vi "Detect Phase.vi"(11 "Input Wavceform":waveform(i16)) -> (1 "Phase in Degress":dbl, 2 "Phase in Samples":dbl, 3 "Detected Sine Frequency":dbl format="%.2p")   [LabVIEW 2011]
uses:
  <vilib>/measure/matone.llb/Extract Single Tone Information 1 Chan.vi
  <vilib>/measure/NI_MAPro.lvlib
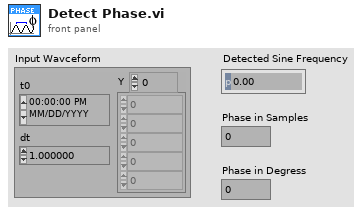
[diagram p1: front panel]
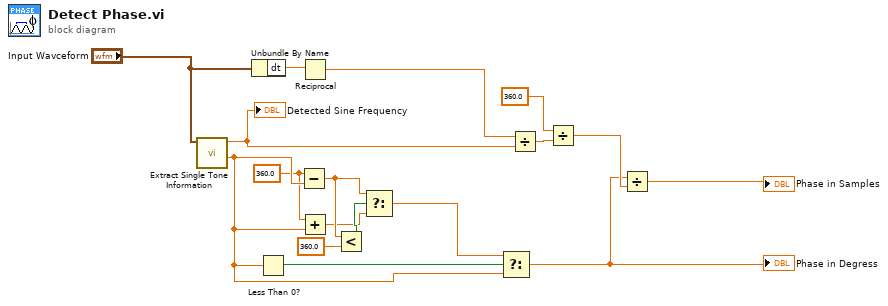
[diagram p0: block diagram]
diagram:
  w5 = 360.0 ("x")
  n1 = call-poly <vilib>:"Extract Single Tone Information.vi"("time signal in"="Input Wavceform") -> ("detected phase (deg)"=w6:dbl, "detected frequency"=w12:dbl)  [unwired: 5 in, 4 out]
  "Detected Sine Frequency" <- w12
  n2 = Unbundle By Name("Input Wavceform") -> ("dt"=w2:dbl)
  n3 = Less Than 0?(x=w6) -> (x < 0?=w4:bool)
  n4 = Subtract(x=w5, y=w6) -> (x-y=w9:dbl)
  n5 = Reciprocal(x=w2) -> (1/x=w1:dbl)
  n6 = Add(x=w5, y=w6) -> (x+y=w7:dbl)
  n7 = Less?(x=w9, y=360.0) -> (x < y?=w8:bool)
  n8 = Select(t=w9, s=w8, f=w7) -> (s? t:f=w11:dbl)
  n9 = Select(t=w11, s=w4, f=w6) -> (s? t:f=w13:dbl)
  "Phase in Degress" <- w13
  n10 = Divide(x=w1, y=w12) -> (x/y=w15:dbl)
  n11 = Divide(x=360.0 ("y"), y=w15) -> (x/y=w14:dbl)
  n12 = Divide(x=w13, y=w14) -> (x/y=→"Phase in Samples":dbl)
